vi "Init Module.vi"(8 "error in (no error)":errorcluster, 11 "Singleton Module Admin in":refnum<class "Delacor_lib_QMH_Module Admin.lvclass">) -> (0 "error out":errorcluster, 2 "Manipulator Request Events":T1, 3 "Singleton Module Admin out":refnum<class "Delacor_lib_QMH_Module Admin.lvclass">)   [LabVIEW 2020, in "Manipulator.lvlib"]
doc: "Initialize the module by creating Broadcast Events, Request Events, and synchronization rendezvous.\n_____\nBased on DQMH Project Template 6.0.0.91."
uses:
  Manipulator.lvlib
  <vilib>/Delacor/Delacor QMH/Libraries/Module Admin_class/Delacor_lib_QMH_Module Admin.lvclass
  Request Events--cluster.ctl
  Stop Argument--cluster.ctl
  Show Panel Argument--cluster.ctl
  Hide Panel Argument--cluster.ctl
  Get Module Execution Status Argument--cluster.ctl
  Show Diagram Argument--cluster.ctl
  Get Num Axes Argument--cluster.ctl
  Get Num Axes (Reply Payload)--cluster.ctl
  Get Position and Speed Argument--cluster.ctl
  Get Position and Speed (Reply Payload)--cluster.ctl
  Move Axis Argument--cluster.ctl
  Move Axis (Reply Payload)--cluster.ctl
  Get Status Argument--cluster.ctl
  Get Status (Reply Payload)--cluster.ctl
  Manipulator-CLIDriver/Manipulator Status.ctl
  Move Axis with Speed Argument--cluster.ctl
  Move Axis with Speed (Reply Payload)--cluster.ctl
  Move to Named Position Argument--cluster.ctl
  Settings/Named Position.ctl
  Move to Named Position (Reply Payload)--cluster.ctl
  Add Named Position Argument--cluster.ctl
  Add Named Position (Reply Payload)--cluster.ctl
  Delete Named Position Argument--cluster.ctl
  Delete Named Position (Reply Payload)--cluster.ctl
  Get Named Positions Argument--cluster.ctl
  Get Named Positions (Reply Payload)--cluster.ctl
  Manipulator-CLIDriver/Manipulator CLI Driver.lvlib
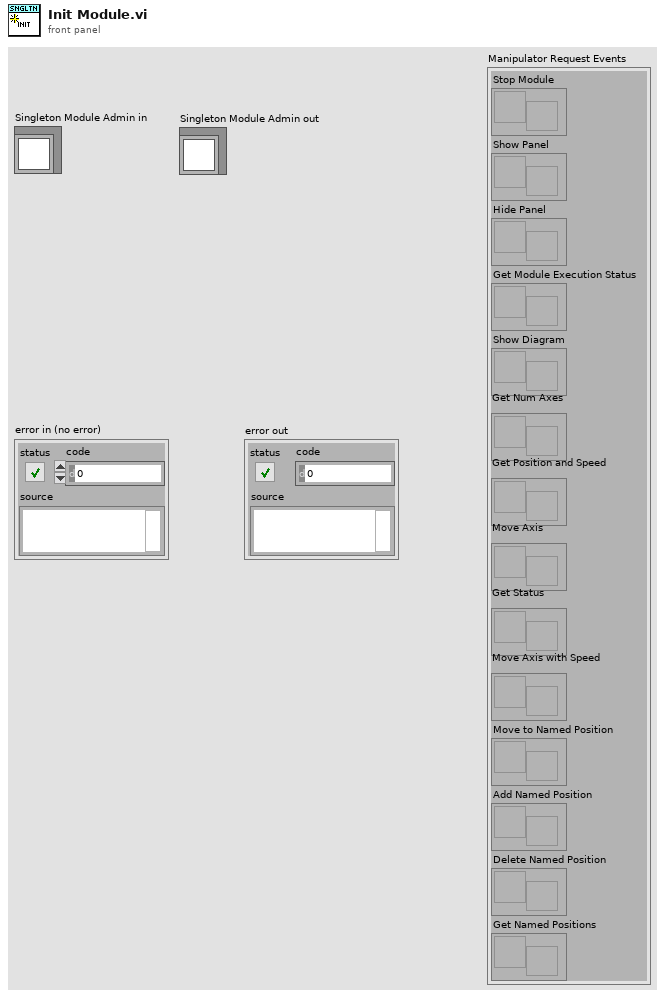
[diagram p1: front panel]
types:
  T1 = typedef "Manipulator.lvlib/Request Events--cluster.ctl" = cluster{"Stop Module":refnum<user-event>, "Show Panel":refnum<user-event>, "Hide Panel":refnum<user-event>, "Get Module Execution Status":refnum<user-event>, "Show Diagram":refnum<user-event>, "Get Num Axes":refnum<user-event>, "Get Position and Speed":refnum<user-event>, "Move Axis":refnum<user-event>, "Get Status":refnum<user-event>, "Move Axis with Speed":refnum<user-event>, "Move to Named Position":refnum<user-event>, "Add Named Position":refnum<user-event>, "Delete Named Position":refnum<user-event>, "Get Named Positions":refnum<user-event>}
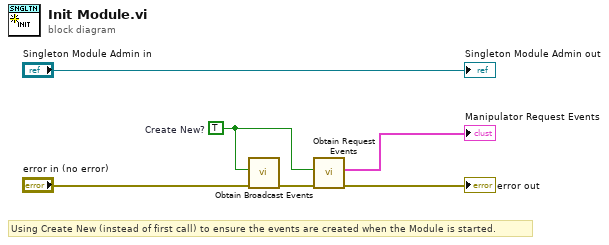
[diagram p0: block diagram]
diagram:
  w3 = TRUE  # Create New?
  # "Using Create New (instead of first call) to ensure the events are created when the Module is started."
  n1 = call "Obtain Broadcast Events.vi"("error in (no error)"="error in (no error)", "Create New? (F)"=w3) -> ("error out"=w6:errorcluster)  [unwired: 8 in, 1 out]
  n2 = call "Obtain Request Events.vi"("error in (no error)"=w6, "Create New? (F)"=w3) -> ("error out"=→"error out":errorcluster, "Manipulator Request Events"=→"Manipulator Request Events":T1)  [unwired: 8 in]
  "Singleton Module Admin out" <- "Singleton Module Admin in"
